vi "Get Param.vi"(3 "error in (no error)":errorcluster, 4 "param":dbl, 5 "paramID":i32) -> (0 "error out":errorcluster, 1 "param out":dbl, 2 "function return":i32)   [LabVIEW 2020, in "ThorConfocal.lvlib"]
doc: "long GetParam(const long paramID, double &param);"
uses:
  ThorConfocal.lvlib
  ThorConfocal.dll
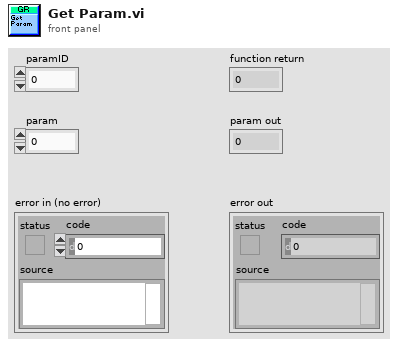
[diagram p1: front panel]
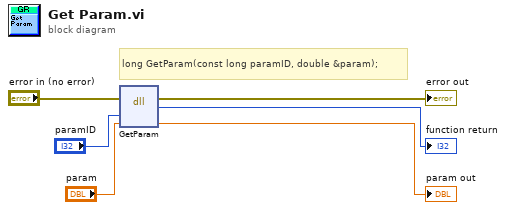
[diagram p0: block diagram]
diagram:
  # "long GetParam(const long paramID, double &param);"
  n1 = dll-call lib="D:/software/TweezerTron/ThorConfocal.dll" fn="GetParam"(error in="error in (no error)", "paramID"="paramID", "param"="param") -> (error out=→"error out":errorcluster, "return type"=→"function return":i32, "param"=→"param out":dbl)  [unwired: 3 in, 1 out]
